vi "Get ni_measurements_v1_MeasurementService_Measure Request.vi"(8 "error in (no error)":errorcluster, 11 "gRPCid in":T1) -> (0 "error out":errorcluster, 2 "Message Data":T2, 3 "gRPCid out":T1)   [LabVIEW 2020, in "Line Regulation.lvlib" / "MeasurementService.lvclass"]
uses:
  MeasurementService.lvclass
  <vilib>/gRPC/LabVIEW gRPC Library/Server API/typeDefs/grpcId.ctl
  RPC Messages/ni_measurements_v1_MeasureRequest.ctl
  RPC Messages/google_protobuf_Any.ctl
  MeasurementService.lvclass/MeasurementService.ctl
  Line Regulation.lvlib
  <vilib>/gRPC/LabVIEW gRPC Library/gprc-lvsupport-release.lvlib
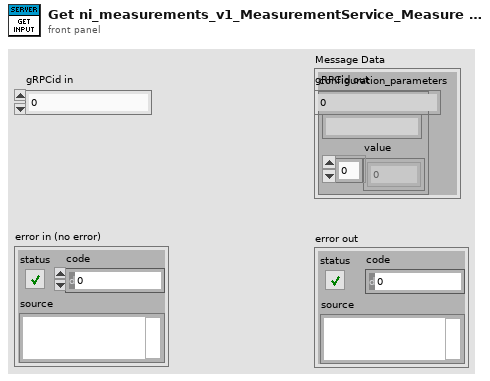
[diagram p1: front panel]
types:
  T1 = typedef "gprc-lvsupport-release.lvlib/grpcId.ctl" = u64
  T2 = typedef "Line Regulation.lvlib/ni_measurements_v1_MeasureRequest.ctl" = cluster{"configuration_parameters":T3}
  T3 = typedef "Line Regulation.lvlib/google_protobuf_Any.ctl" = cluster{"type_url":string, "value":u8[]}
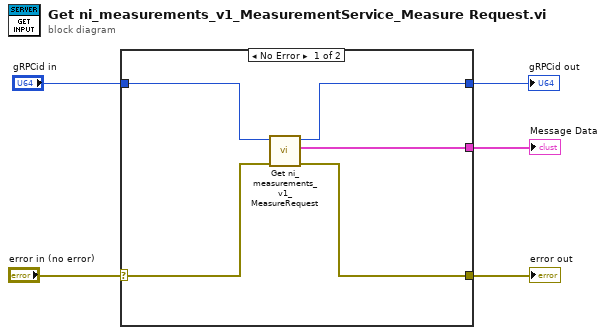
[diagram p0: block diagram]
diagram:
  n1 = case shown="No Error" "error in (no error)" {
    selector: "error in (no error)" -> [w10 w11]
    tunnel: [w9 w11] -> w4
    tunnel: "gRPCid in" -> [w8 w12]
    tunnel: [w7 _] -> w2
    tunnel: [w6 w12] -> w1
    frame No Error {
      n2 = call "Get ni_measurements_v1_MeasureRequest.vi"("error in (no error)"=w10, "gRPCid"=w8) -> ("error out"=w9:errorcluster, "package_templatemessage"=w7:T2, "gRPCid out"=w6:T1)  [unwired: 7 in]
    }
    frame Error {
    }
  }
  "error out" <- w4
  "Message Data" <- w2
  "gRPCid out" <- w1
